vi "Detect Peaks from Waveform.vi"(8 "Error In":errorcluster, 9 "Peak Threshold":dbl, 10 "Peak Width":dbl, 11 "Normalized Waveform In":waveform(dbl)) -> (0 "dt(sec)":dbl, 2 "Peak Amplitudes":dbl[](array[numeric]), 3 "Peak Locations":dbl[](array[numeric]), 4 "Valid Peaks Found?":bool, 6 "Error Out":errorcluster)   [LabVIEW 2025]
uses:
  <vilib>/Analysis/NI_AAL_SigProc.lvlib
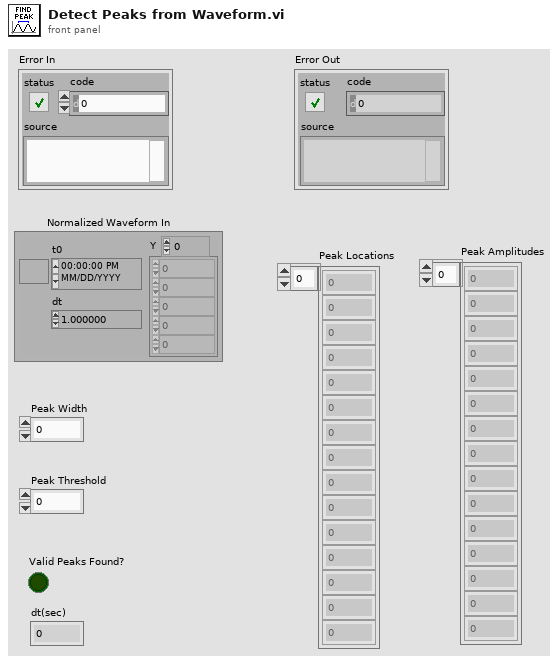
[diagram p1: front panel]
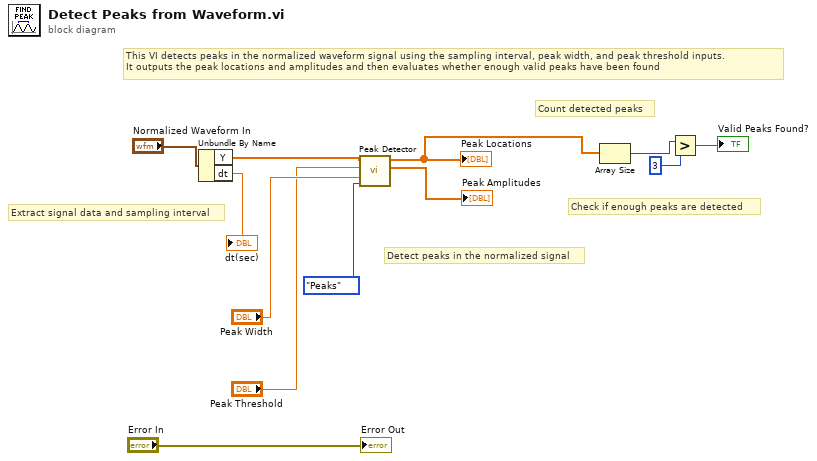
[diagram p0: block diagram]
diagram:
  # "Count detected peaks"
  # "Check if enough peaks are detected"
  # "Detect peaks in the normalized signal"
  # "Extract signal data and sampling interval"
  # "This VI detects peaks in the normalized waveform signal using the sampling interval, peak width, and peak threshold inputs. \nIt outputs the peak locations and amplitudes and then evaluates whether enough valid peaks have been found"
  n1 = Unbundle By Name("Normalized Waveform In") -> ("Y"=w10:dbl[], "dt"=→"dt(sec)":dbl)
  n2 = call <vilib>:"Peak Detector.vi"("peaks/valleys"=enum32{"Peaks", "Valleys"}."Peaks", "width"="Peak Width", "threshold"="Peak Threshold", "X"=w10) -> ("Amplitudes"=→"Peak Amplitudes":dbl[], "Locations"=w5:dbl[])  [unwired: 3 in, 3 out]
  "Peak Locations" <- w5
  n3 = Array Size(array=w5) -> (size(s)=w4:i32)
  n4 = Greater?(x=w4, y=3) -> (0:→"Valid Peaks Found?":bool)
  "Error Out" <- "Error In"
